vi "TDMS Write.vi"(7 "Channel Name":string, 8 "error in (no error)":errorcluster, 9 "Group Name":string, 10 "TDMS in":refnum<k34>, 11 "Enum in":refnum<class "Enum.lvclass">) -> (0 "error out":errorcluster, 2 "TDMS Out":refnum<k34>)   [LabVIEW 2020, in "Data.lvlib" / "Enum.lvclass"]
doc: "Write Generic Data to a TDMS file.\nThis implementation writes the Enum index with 'Channel Name' and the Enum Alias as 'Channel Name'_Alias."
uses:
  Enum.lvclass
  Enum.lvclass/Enum.ctl
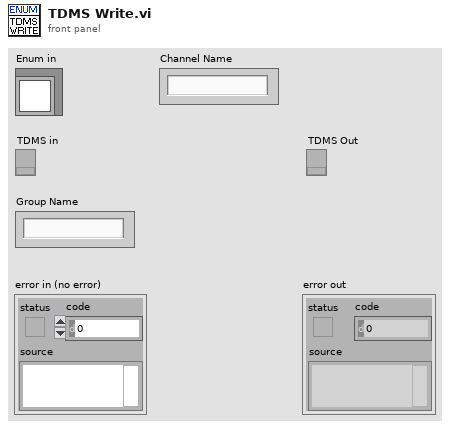
[diagram p1: front panel]
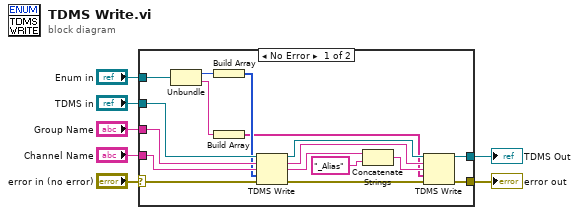
[diagram p0: block diagram]
diagram:
  n1 = case shown="No Error" "error in (no error)" {
    selector: "error in (no error)" -> [w24 w25]
    tunnel: [w16 w25] -> w2
    tunnel: "TDMS in" -> [w22 w26]
    tunnel: [w14 w26] -> w1
    tunnel: "Channel Name" -> [w21 _]
    tunnel: "Group Name" -> [w20 _]
    tunnel: "Enum in" -> [w19 _]
    frame No Error {
      n2 = Unbundle(w19) -> (w18:u32, w9:string)
      n3 = Build Array(w18) -> (w17:u32[])
      n4 = Build Array(w9) -> (w8:string[])
      n5 = TDMS Write(0:w22, 5:w20, 7:w21, 9:w17, 11:w24) -> (4:w15:refnum<k34>, 6:w13:string, 8:w12:string, 15:w23:errorcluster)  [unwired: 1 in]
      n6 = Concatenate Strings(w12, "_Alias" ("string")) -> (w10:string)
      n7 = TDMS Write(0:w15, 5:w13, 7:w10, 9:w8, 11:w23) -> (4:w14:refnum<k34>, 15:w16:errorcluster)  [unwired: 1 in, 2 out]
    }
    frame Error {
    }
  }
  "error out" <- w2
  "TDMS Out" <- w1
